vi "Clock Generalization.vi"() -> ()   [LabVIEW 2020]
uses:
  Global Parameters.vi
panel:
  out "Actual Duty Cycle":dbl=0.5
  out "Actual Frequency":dbl=1000.0
  out "Duty Cycle":dbl=0.5 format="%.6f"
  out "Frequency":dbl=1000.0 format="%.6f"
  out "Output Terminal":tag="/Dev1/PFI2"
  out "Counter":tag="Dev1/ctr0"
  in  "Clock Open":bool
  # "Please light up this indicator before running"
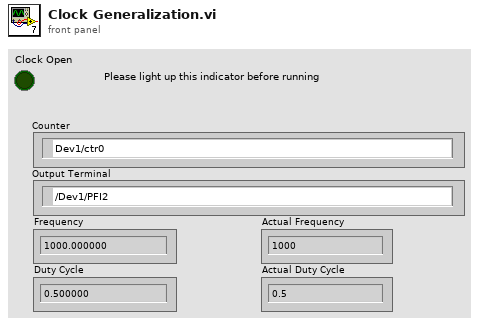
[diagram p1: front panel]
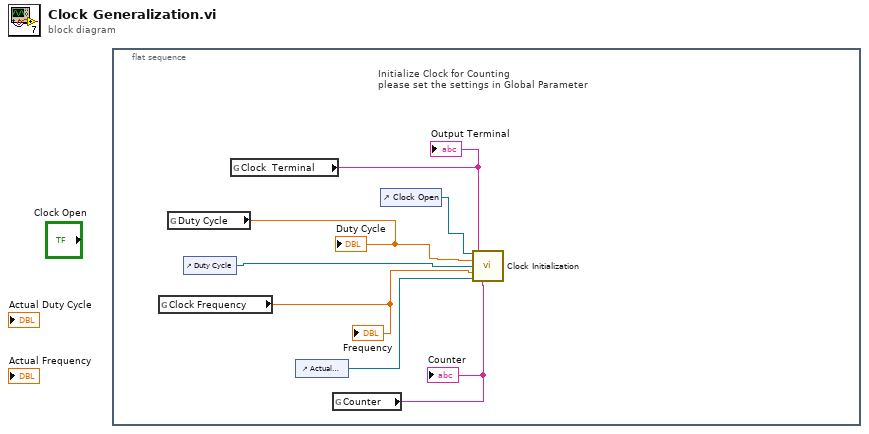
[diagram p0: block diagram]
diagram:
  n1 = flat-sequence {
    frame #0 {
      # "Initialize Clock for Counting\nplease set the settings in Global Parameter"
      n2 = global read "Global Parameters.vi" "Clock Frequency"() -> (w5:dbl)
      "Frequency" <- w5
      n3 = global read "Global Parameters.vi" "Duty Cycle"() -> (w3:dbl)
      "Duty Cycle" <- w3
      n4 = control-ref of="Duty Cycle"() -> (w4:refnum<vi>)
      n5 = global read "Global Parameters.vi" "Clock  Terminal"() -> (w7:tag)
      "Output Terminal" <- w7
      n6 = control-ref of="Actual Frequency"() -> (w1:refnum<vi>)
      n7 = global read "Global Parameters.vi" "Counter"() -> (w6:tag)
      "Counter" <- w6
      n8 = control-ref of="Clock Open"() -> (w2:refnum<vi>)
      n9 = call "Clock Initialization.vi"("Boolean in"=w2, "Output Terminal"=w7, "Duty Cycle"=w3, "Actual Duty Cycle"=w4, "Frequency"=w5, "Actual Frequency"=w1, "Counter"=w6) -> ()  [unwired: 9 in]
    }
  }
